vi "Reset all channels.vi"(8 "Error In":errorcluster, 11 "Arduino Port":refnum<visa-resource-name>) -> (0 "Error Out":errorcluster, 3 "Arduino Port out":refnum<visa-resource-name>)   [LabVIEW 2016]
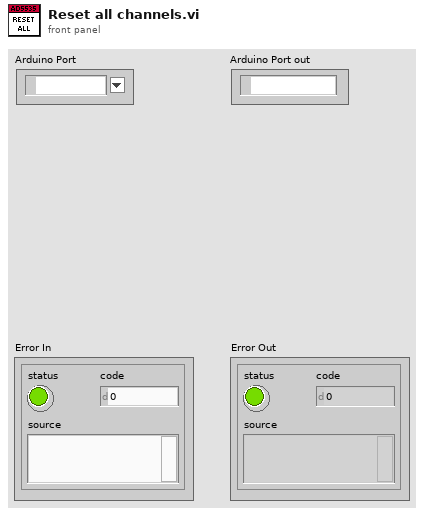
[diagram p1: front panel]
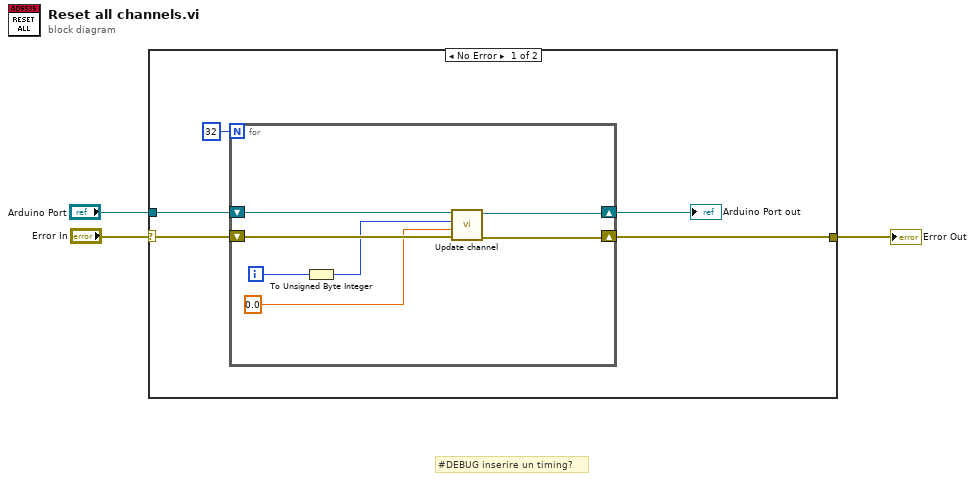
[diagram p0: block diagram]
diagram:
  # "#DEBUG inserire un timing?"
  n1 = case shown="No Error" "Error In" {
    selector: "Error In" -> [w7 w16]
    tunnel: [w6 w16] -> w2
    tunnel: "Arduino Port" -> [w8 _]
    frame No Error {
      n2 = for {
        N: 32 -> [_]
        shift-right: [w13] -> w5
        shift-left: w8 -> [w14]
        shift-right: [w11] -> w6
        shift-left: w7 -> [w12]
        i -> [w15]
        n3 = To Unsigned Byte Integer(number=w15) -> (unsigned 8bit integer=w10:u8)
        n4 = call "Update channel.vi"("Error In"=w12, "Value"=sgl 0.0, "Channel"=w10, "Arduino Port"=w14) -> ("Error Out"=w11:errorcluster, "Arduino Port out"=w13:refnum<visa-resource-name>)  [unwired: 6 in]
      }
      "Arduino Port out" <- w5
    }
    frame Error {
    }
  }
  "Error Out" <- w2
